vi "InitialFile.vi"(8 "UTC format":bool, 9 "Extension":string, 10 "PreAppend Name":string, 11 "Base Path":path) -> (3 "File Path":path)   [LabVIEW 2015]
doc: "From the base path, Pre-append name and extension, finds a unique file name: PreYYYYMMDDxnnn.ext. If the directory PreYYYYMMDD does not exist in the base path, it is created.\n\nLA Watts 20100505"
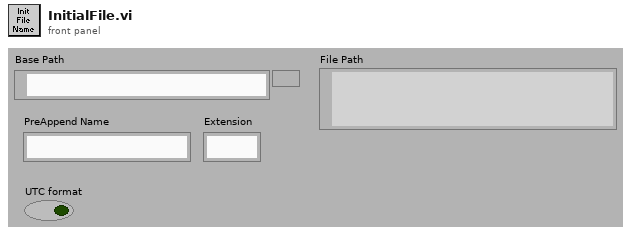
[diagram p1: front panel]
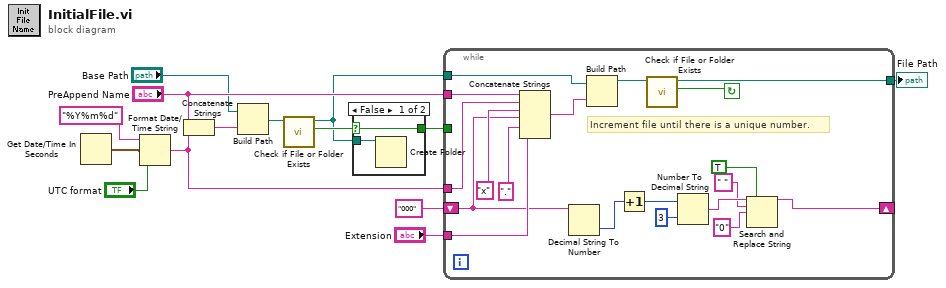
[diagram p0: block diagram]
diagram:
  n1 = Get Date/Time In Seconds() -> (seconds since 1Jan1904=w13:timestamp)
  n2 = Format Date/Time String(time format string (%c)="%Y%m%d", seconds (now)=w13, UTC format="UTC format") -> (date/time string=w8:string)
  n3 = Concatenate Strings("PreAppend Name", w8) -> (w7:string)
  n4 = Build Path(base path="Base Path", name or relative path=w7) -> (appended path=w5:path)
  n5 = call <vilib>:"Check if File or Folder Exists.vi"("path"=w5) -> ("file or folder exists?"=w4:bool, "dup path"=w1:path)  [unwired: 8 in, 1 out]
  n6 = case shown="False" w4 {
    selector: w4 -> [w15 w17]
    tunnel: w1 -> [w16 _]
    tunnel: [w15 w17] -> w3
    frame False {
      n7 = Create Folder(path (use dialog)=w16) -> ()  [unwired: 2 in, 3 out]
    }
    frame True {
    }
  }
  n8 = while {
    tunnel: w8 -> [w35]
    tunnel: "PreAppend Name" -> [w36]
    tunnel: "Extension" -> [w32]
    shift-right: [w18] -> _
    shift-left: "000" -> [w30]
    tunnel: w3 -> [_]
    tunnel: [w24] -> w2
    tunnel: w1 -> [w23]
    stop <- w26 continue-if-true
    # "Increment file until there is a unique number."
    n9 = Concatenate Strings(w36, w35, "x", w30, ".", w32) -> (w31:string)
    n10 = Decimal String To Number(string=w30) -> (number=w29:i32)  [unwired: 2 in, 1 out]
    n11 = Build Path(base path=w23, name or relative path=w31) -> (appended path=w27:path)
    n12 = Increment(x=w29) -> (x+1=w28:i32)
    n13 = call <vilib>:"Check if File or Folder Exists.vi"("path"=w27) -> ("file or folder exists?"=w26:bool, "dup path"=w24:path)  [unwired: 8 in, 1 out]
    n14 = Number To Decimal String(number=w28, width (-)=i16 3) -> (decimal integer string=w22:string)
    n15 = Search and Replace String(replace all?=TRUE ("replace all? (F)"), input string=w22, search string=" ", replace string="0" ("replace string (\"\")")) -> (result string=w18:string)  [unwired: 4 in, 3 out]
  }
  "File Path" <- w2
